vi "重测.vi"(9 "Last SN":string, 10 "DBSet":T1, 11 "SN":string) -> (0 "继续?":bool, 1 "重测？":bool, 3 "重测原因":string)   [LabVIEW 2011]
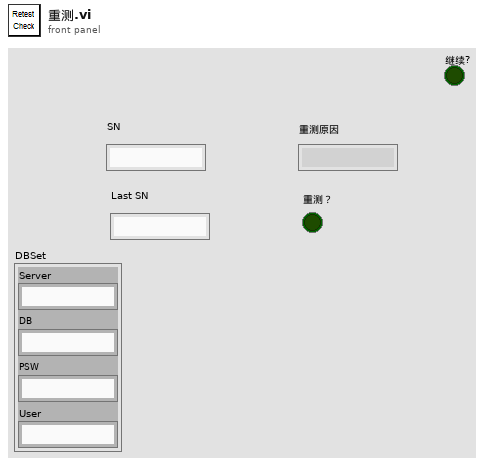
[diagram p1: front panel]
types:
  T1 = cluster{"Server":string, "DB":string, "PSW":string, "User":string}
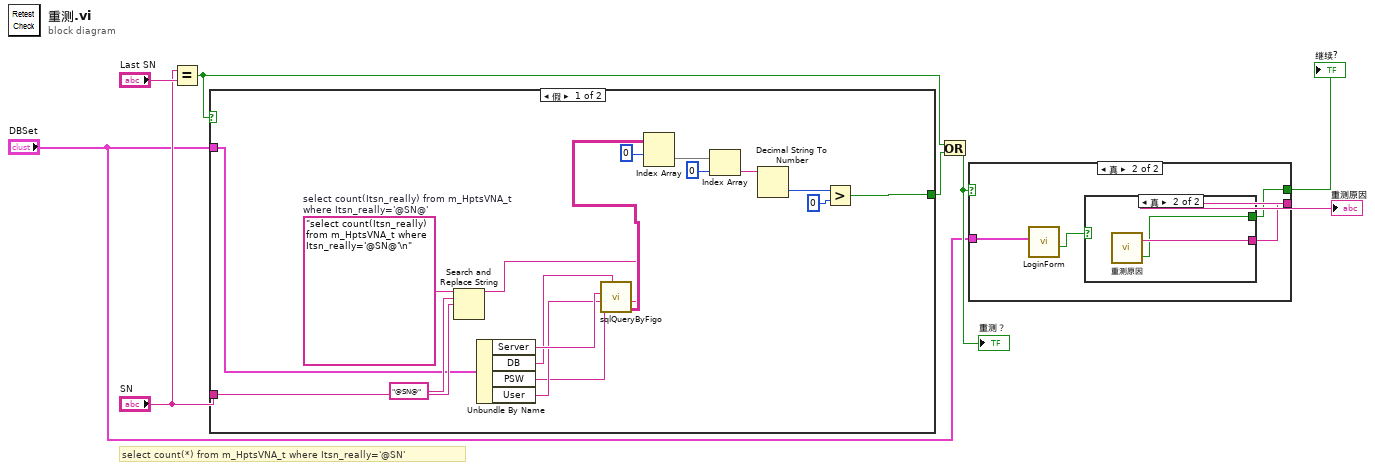
[diagram p0: block diagram]
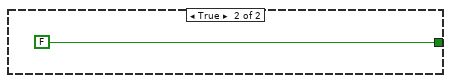
[diagram p2: hidden frame]
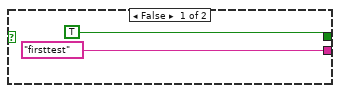
[diagram p3: hidden frame]
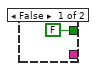
[diagram p4: hidden frame]
diagram:
  # "select count(*) from m_HptsVNA_t where Itsn_really='@SN'"
  n1 = Equal?(x="SN", y="Last SN") -> (x = y?=w5:bool)
  n2 = case shown="假" w5 {
    tunnel: "SN" -> [w23 _]
    tunnel: [w16 FALSE] -> w6
    tunnel: "DBSet" -> [w15 _]
    frame False {
      w24 = "select count(Itsn_really) from m_HptsVNA_t where Itsn_really='@SN@'\n"  # select count(Itsn_really) from m_HptsVNA_t where Itsn_really='@SN@'
      n3 = Search and Replace String(input string=w24, search string="@SN@" ("搜索字符串"), replace string=w23) -> (result string=w13:string)  [unwired: 5 in, 3 out]
      n4 = Unbundle By Name(w15) -> ("Server"=w12:string, "DB"=w11:string, "PSW"=w9:string, "User"=w10:string)
      n5 = call "sqlQueryByFigo.vi"("SQL"=w13, "DATABASE"=w11, "password"=w9, "user id"=w10, "Server"=w12) -> ("查询数据"=w14:string[][])  [unwired: 5 in, 1 out]
      n6 = Index Array(array=w14, index (row)=0 ("索引 (行)")) -> (element=w21:string[])  [unwired: 1 in]
      n7 = Index Array(array=w21, index=0 ("索引")) -> (element=w19:string)
      n8 = Decimal String To Number(string=w19) -> (number=w18:i32)  [unwired: 2 in, 1 out]
      n9 = Greater?(x=w18, y=0) -> (0:w16:bool)
    }
    frame True {
    }
  }
  n10 = Or(x=w5, y=w6) -> (x .or. y?=w4:bool)
  "重测？" <- w4
  n11 = case shown="真" w4 {
    tunnel: ["firsttest" ("重测原因") w32] -> w3
    tunnel: [TRUE ("继续?") w31] -> w2
    tunnel: "DBSet" -> [_ w30]
    frame False {
    }
    frame True {
      n12 = call "LoginForm.vi"("DBSet"=w30) -> ("登录成功"=w29:bool)  [unwired: 2 out]
      n13 = case shown="真" w29 {
        tunnel: [_ w35] -> w32
        tunnel: [FALSE ("继续?") w34] -> w31
        frame False {
        }
        frame True {
          n14 = call "重测原因.vi"() -> ("重测原因str"=w35:string, "继续"=w34:bool)  [unwired: 1 in]
        }
      }
    }
  }
  "重测原因" <- w3
  "继续?" <- w2
